vi "ToDatagram.vi"(8 "error in (no error)":errorcluster, 10 "messageID":u16, 11 "PingMqttMsg in":refnum<class "PingMqttMsg.lvclass">) -> (0 "error out":errorcluster, 2 "Datagram":u8[](array[numeric]), 3 "PingMqttMsg out":refnum<class "PingMqttMsg.lvclass">)   [LabVIEW 2020, in "PingMqttMsg.lvclass"]
uses:
  PingMqttMsg.lvclass
  mqttTypedef/MessageType.ctl
  mqttTypedef/QosLevel.ctl
  BaseMqttMsg.lvclass
  MQTT Client.lvclass
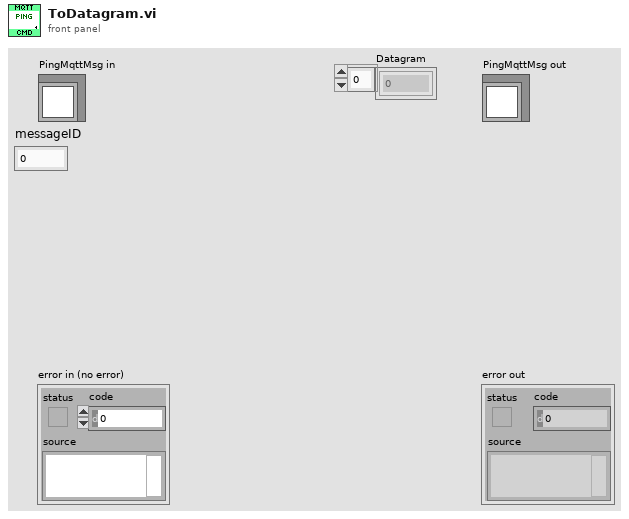
[diagram p1: front panel]
types:
  T1 = typedef "MQTT Client.lvclass/QosLevel.ctl" = enum8{"At most once", "At least once", "Exactly once", "Reserved"}
  T2 = typedef "MQTT Client.lvclass/MessageType.ctl" = enum32{"Reserved", "CONNECT", "CONNACK", "PUBLISH", "PUBACK", "PUBREC", "PUBREL", "PUBCOMP", "SUBSCRIBE", "SUBACK", "UNSUBSCRIBE", "UNSUBACK", "PINGREQ", "PINGRESP", "DISCONNECT", "Reserved2"}
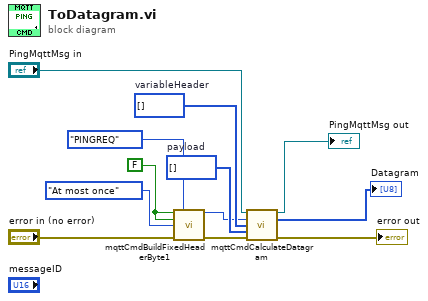
[diagram p0: block diagram]
diagram:
  w11 = u8[] []  # payload
  w10 = u8[] []  # variableHeader
  w8 = FALSE ("retain(F)")
  n1 = call "mqttCmdBuildFixedHeaderByte1.vi"("retain(F)"=w8, "MessageType"=MessageType."PINGREQ", "duplicate(F)"=w8, "QoS (At most once)"=QosLevel."At most once", "error in (no error)"="error in (no error)") -> ("byte1"=w9:u8, "error out"=w12:errorcluster)  [unwired: 9 in]
  n2 = call-dynamic "mqttCmdCalculateDatagram.vi"("mqttCmd in"="PingMqttMsg in", "FixedHeaderByte1"=w9, "variableHeader"=w10, "payload"=w11, "error in (no error)"=w12) -> ("mqttCmd out"=→"PingMqttMsg out":refnum<class "PingMqttMsg.lvclass">, "Datagram"=→"Datagram":u8[], "error out"=→"error out":errorcluster)  [unwired: 8 in]
